vi "DROPBEAR_Model_Updating_Postprocessing.vi"(8 "error in (no error)":errorcluster, 11 "DROPBEAR_Model_Updating in":refnum<class "DROPBEAR_Model_Updating.lvclass">) -> (0 "Cycle time":dbl, 1 "Nodal":dynamicdata(graph), 2 "Meter":dynamicdata(graph), 3 "Frequency":dynamicdata(graph))   [LabVIEW 2021, in "DROPBEAR_Model_Updating.lvclass"]
uses:
  DROPBEAR_Model_Updating.lvclass
  DROPBEAR_Model_Updating.lvclass/DROPBEAR_Model_Updating.ctl
  Data_Array/Data_Array.lvclass
panel:
  out "Waveform Graph 2":dbl[](graph)
  out "Waveform Graph":dbl[](graph)
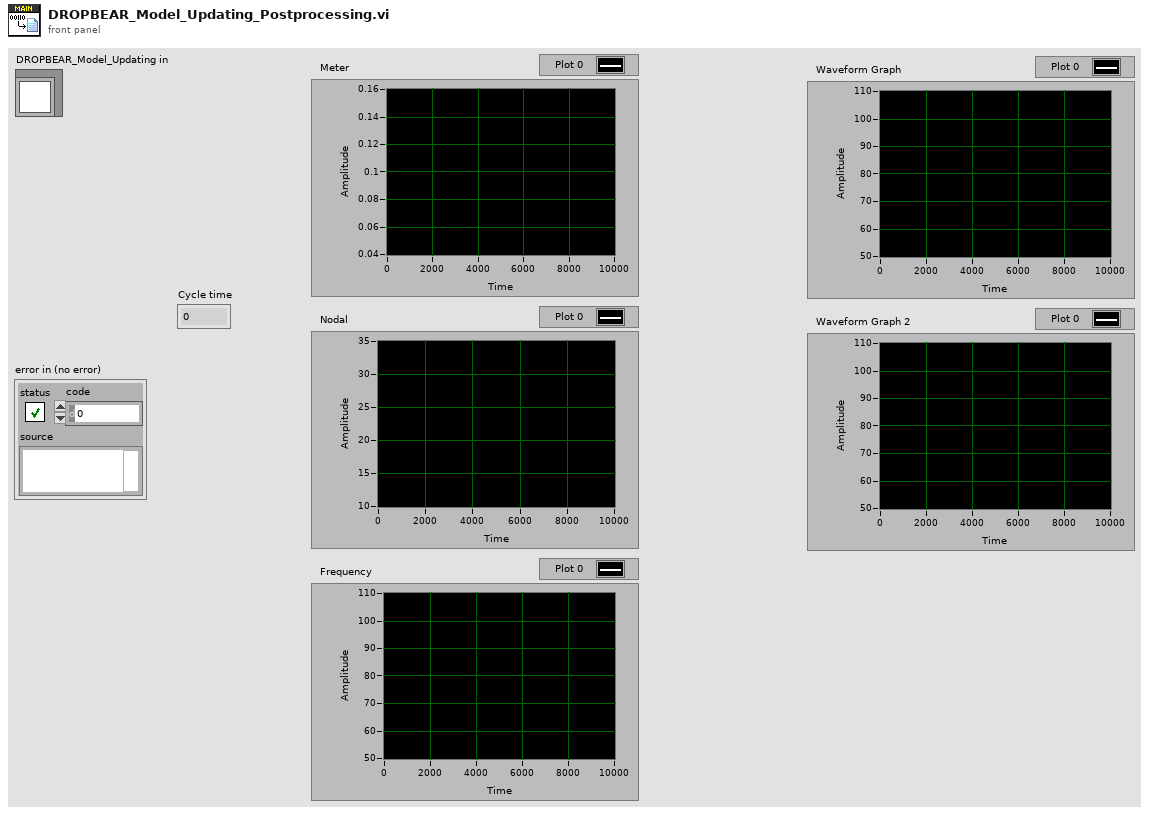
[diagram p1: front panel]
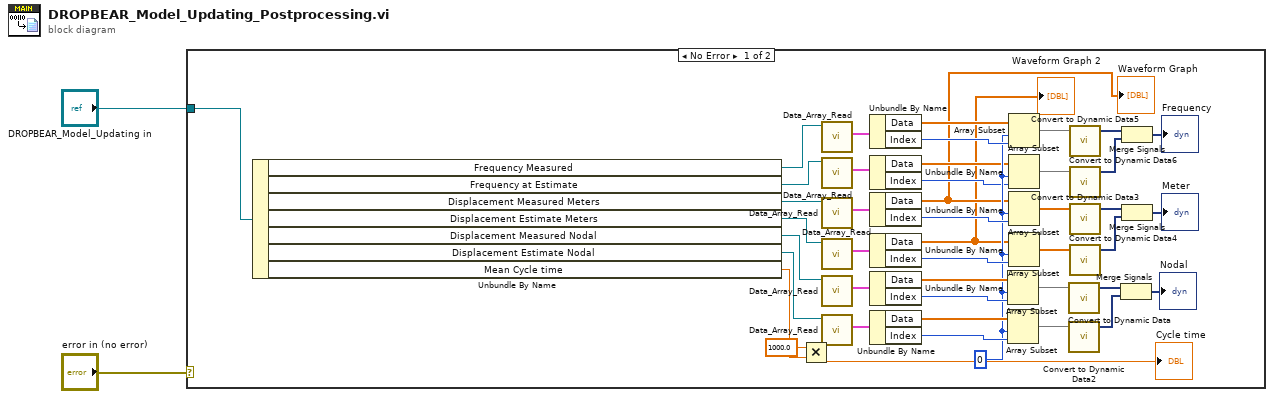
[diagram p0: block diagram]
diagram:
  n1 = case shown="No Error" "error in (no error)" {
    tunnel: "DROPBEAR_Model_Updating in" -> [w46 _]
    frame No Error {
      w14 = 0 ("index")
      n2 = Unbundle By Name(w46) -> ("Frequency Measured"=w13:refnum<class "Data_Array.lvclass">, "Frequency at Estimate"=w12:refnum<class "Data_Array.lvclass">, "Displacement Measured Meters"=w26:refnum<class "Data_Array.lvclass">, "Displacement Estimate Meters"=w27:refnum<class "Data_Array.lvclass">, "Displacement Measured Nodal"=w45:refnum<class "Data_Array.lvclass">, "Displacement Estimate Nodal"=w44:refnum<class "Data_Array.lvclass">, "Mean Cycle time"=w43:dbl)
      n3 = Multiply(x=1000.0, y=w43) -> (x*y=→"Cycle time":dbl)
      n4 = call-dynamic "Data_Array_Read.vi"("Data_Array in"=w13) -> ("Data_params"=w10:cluster{"Data":dbl[], "Index":i32, "Buffer":i32})  [unwired: 8 in, 2 out]
      n5 = call-dynamic "Data_Array_Read.vi"("Data_Array in"=w12) -> ("Data_params"=w11:cluster{"Data":dbl[], "Index":i32, "Buffer":i32})  [unwired: 8 in, 2 out]
      n6 = call-dynamic "Data_Array_Read.vi"("Data_Array in"=w26) -> ("Data_params"=w25:cluster{"Data":dbl[], "Index":i32, "Buffer":i32})  [unwired: 8 in, 2 out]
      n7 = call-dynamic "Data_Array_Read.vi"("Data_Array in"=w27) -> ("Data_params"=w24:cluster{"Data":dbl[], "Index":i32, "Buffer":i32})  [unwired: 8 in, 2 out]
      n8 = call-dynamic "Data_Array_Read.vi"("Data_Array in"=w45) -> ("Data_params"=w33:cluster{"Data":dbl[], "Index":i32, "Buffer":i32})  [unwired: 8 in, 2 out]
      n9 = call-dynamic "Data_Array_Read.vi"("Data_Array in"=w44) -> ("Data_params"=w34:cluster{"Data":dbl[], "Index":i32, "Buffer":i32})  [unwired: 8 in, 2 out]
      n10 = Unbundle By Name(w10) -> ("Data"=w6:dbl[], "Index"=w17:i32)
      n11 = Unbundle By Name(w11) -> ("Data"=w5:dbl[], "Index"=w9:i32)
      n12 = Unbundle By Name(w25) -> ("Data"=w4:dbl[], "Index"=w30:i32)
      "Waveform Graph" <- w4
      n13 = Unbundle By Name(w24) -> ("Data"=w3:dbl[], "Index"=w29:i32)
      "Waveform Graph 2" <- w3
      n14 = Unbundle By Name(w33) -> ("Data"=w37:dbl[], "Index"=w40:i32)
      n15 = Unbundle By Name(w34) -> ("Data"=w36:dbl[], "Index"=w39:i32)
      n16 = Array Subset(array=w37, index=w14, length=w40) -> (w38:dbl[])
      n17 = Array Subset(array=w36, index=w14, length=w39) -> (w35:dbl[])
      n18 = Array Subset(array=w6, index=w14, length=w17) -> (w16:dbl[])
      n19 = Array Subset(array=w5, index=w14, length=w9) -> (w8:dbl[])
      n20 = Array Subset(array=w4, index=w14, length=w30) -> (w28:dbl[])
      n21 = Array Subset(array=w3, index=w14, length=w29) -> (w7:dbl[])
      n22 = call "Convert to Dynamic Data"("Array"=w38) -> ("Dynamic Data Type"=w42:dynamicdata)  [unwired: 3 in]
      n23 = call "Convert to Dynamic Data2"("Array"=w35) -> ("Dynamic Data Type"=w41:dynamicdata)  [unwired: 3 in]
      n24 = call "Convert to Dynamic Data5"("Array"=w16) -> ("Dynamic Data Type"=w19:dynamicdata)  [unwired: 3 in]
      n25 = call "Convert to Dynamic Data6"("Array"=w8) -> ("Dynamic Data Type"=w18:dynamicdata)  [unwired: 3 in]
      n26 = call "Convert to Dynamic Data3"("Array"=w28) -> ("Dynamic Data Type"=w32:dynamicdata)  [unwired: 3 in]
      n27 = call "Convert to Dynamic Data4"("Array"=w7) -> ("Dynamic Data Type"=w31:dynamicdata)  [unwired: 3 in]
      n28 = Merge Signals(w42, w41) -> (→"Nodal":dynamicdata)
      n29 = Merge Signals(w19, w18) -> (→"Frequency":dynamicdata)
      n30 = Merge Signals(w32, w31) -> (→"Meter":dynamicdata)
    }
    frame Error {
    }
  }
